vi "Write epochPM_Yr.vi"(8 "error in (no error)":errorcluster, 10 "epochPM_Yr":dbl=2009.0 min=1850.0 max=2100.0, 11 "ProperMotion in":refnum<class "ProperMotion.lvclass">) -> (0 "error out":errorcluster, 3 "ProperMotion out":refnum<class "ProperMotion.lvclass">)   [LabVIEW 2022 SP3, in "TCSDataDefinitions.lvlib" / "TCSCommand.lvlib" / "TargetConfiguration.lvlib" / "Target.lvlib" / "FixedTarget.lvlib" / "ProperMotion.lvclass"]
uses:
  ProperMotion.lvclass
  ProperMotion.lvclass/ProperMotion.ctl
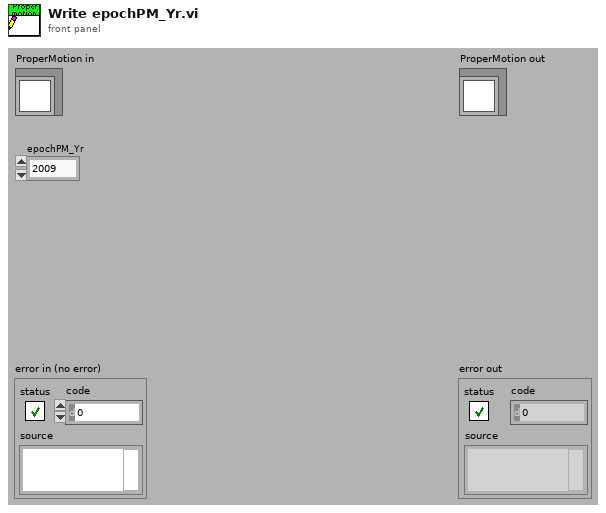
[diagram p1: front panel]
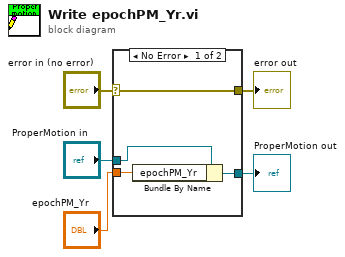
[diagram p0: block diagram]
diagram:
  n1 = case shown="No Error" "error in (no error)" {
    selector: "error in (no error)" -> [w9 w10]
    tunnel: [w9 w10] -> w4
    tunnel: [w7 w11] -> w2
    tunnel: "ProperMotion in" -> [w8 w11]
    tunnel: "epochPM_Yr" -> [w6 _]
    frame No Error {
      n2 = Bundle By Name(cluster=w8, "epochPM_Yr"=w6) -> (w7:refnum<class "ProperMotion.lvclass">)
    }
    frame Error {
    }
  }
  "error out" <- w4
  "ProperMotion out" <- w2
